vi "Error Check Columns.vi"(8 "error in (no error)":errorcluster, 10 "Columns in":refnum<class "Column.lvclass">[](array[class]), 11 "PTS-via-PB in":refnum<class "PTS-via-PB.lvclass">) -> (0 "error out":errorcluster, 2 "Columns OK":bool, 3 "PTS-via-PB out":refnum<class "PTS-via-PB.lvclass">)   [LabVIEW 2013, in "PTS-via-PB.lvclass"]
uses:
  PTS-via-PB.lvclass
  ColumnVIs/Column/Column.lvclass
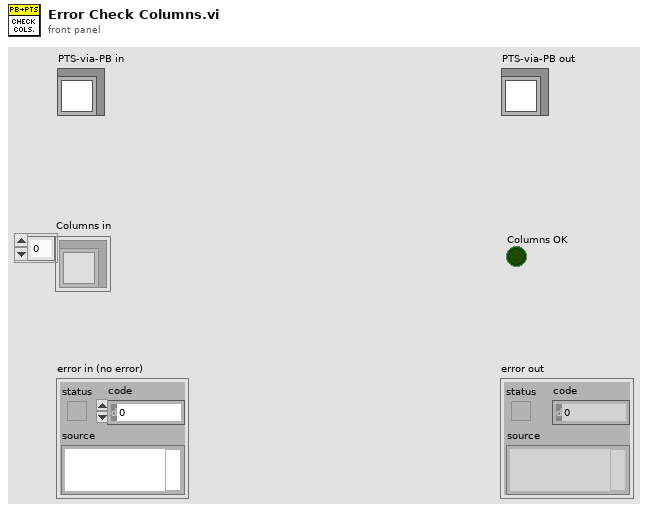
[diagram p1: front panel]
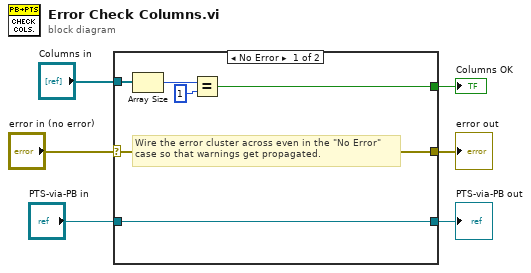
[diagram p0: block diagram]
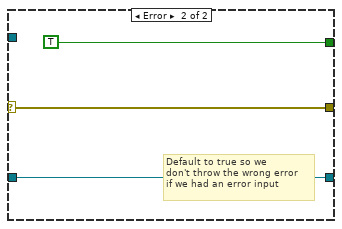
[diagram p2: hidden frame]
diagram:
  n1 = case shown="No Error" "error in (no error)" {
    selector: "error in (no error)" -> [w11 w15]
    tunnel: [w11 w15] -> w2
    tunnel: [w12 w14] -> w4
    tunnel: "PTS-via-PB in" -> [w12 w14]
    tunnel: "Columns in" -> [w8 _]
    tunnel: [w7 TRUE] -> w3
    frame No Error {
      # "Wire the error cluster across even in the \"No Error\"\ncase so that warnings get propagated."
      n2 = Array Size(array=w8) -> (size(s)=w10:i32)
      n3 = Equal?(x=w10, y=1) -> (x = y?=w7:bool)
    }
    frame Error {
      # "Default to true so we\ndon't throw the wrong error\nif we had an error input"
    }
  }
  "error out" <- w2
  "PTS-via-PB out" <- w4
  "Columns OK" <- w3
